vi "ilc.vi"() -> ()   [LabVIEW 2015]
uses:
  Common_RT_ILC/DataTypes/ILCTelemetry.ctl
  Common_RT_ILC/DataTypes/ILCResponses.ctl
  Common_RT_Modbus/DataTypes/ExceptionCodes.ctl
  Common_RT_HPILC/DataTypes/HPResponses.ctl
  Common_RT_HPILC/DataTypes/HPTelemetry.ctl
  Common_RT_HealthAndStatus/RTHealthAndStatus/RTHealthAndStatus.lvclass
  MyHealthAndStatusReadFIFO/MyHealthAndStatusReadFIFO.lvclass
  MyHealthAndStatusWriteFIFO/MyHealthAndStatusWriteFIFO.lvclass
  ModbusFactory/ModbusFactory.lvclass
  SubnetFactory/SubnetFactory.lvclass
  Subnet/DataTypes/SubnetSettings.ctl
  Common_RT_HPILC/DataTypes/HPSettings.ctl
  Common_RT_ILC/DataTypes/ILCSettings.ctl
  Common_RT_Modbus/IModbusFactory/IModbusFactory.lvclass
  ModbusFactory/ModbusFactory.lvclass/ModbusFactory.ctl
  MyHealthAndStatusWriteFIFO/MyHealthAndStatusWriteFIFO.lvclass/MyHealthAndStatusWriteFIFO.ctl
  MyHealthAndStatusReadFIFO/MyHealthAndStatusReadFIFO.lvclass/MyHealthAndStatusReadFIFO.ctl
  Common_RT_HealthAndStatus/RTHealthAndStatus/RTHealthAndStatus.lvclass/RTHealthAndStatus.ctl
  Subnet/Subnet.lvclass/Subnet.ctl
  Common_RT_ILC/ILC/ILC.lvclass/ILC.ctl
  Common_RT_HPILC/HPILC/HPILC.lvclass/HPILC.ctl
  <vilib>/FPGAPlugInAG/cRIO-9038/niLvFpga_Open_cRIO-9038.vi
  <vilib>/rvi/interface/common/dynamic/niFpgaDynamicAddResources.vi
  <vilib>/FPGAPlugInAG/Dynamic/niLvFpga_Abort_Dynamic.vi
  <vilib>/FPGAPlugInAG/Dynamic/niLvFpga_Reset_Dynamic.vi
  <vilib>/FPGAPlugInAG/Dynamic/niLvFpga_Run_Dynamic.vi
  <vilib>/Utility/error.llb/Error Cluster From Error Code.vi
  <vilib>/rvi/errors/niLvFpgaAdjustHostInterfaceError.vi
  <vilib>/FPGAPlugInAG/Dynamic/niLvFpga_Close_Dynamic.vi
  <vilib>/rvi/interface/nirviOpenFPGA/nirviOpenFPGA.xnode
  FPGA Bitfiles/modbus1Port.lvbitx
  FPGA/main.vi
  <vilib>/rvi/interface/nirviMethod/nirviMethod.xnode
  <vilib>/rvi/interface/nirviCloseFPGA/nirviCloseFPGA.xnode
  Common_RT_ILC/RTILC.lvlib
  Common_RT_ILC/ILC/ILC.lvclass
  Common_RT_HPILC/RTHPILC.lvlib
  Common_RT_HPILC/HPILC/HPILC.lvclass
  Common_RT_Modbus/RTModbus.lvlib
  Subnet/Subnet.lvclass
  <vilib>/rvi/errors/niLvFpgaMergeErrorWithErrorCode.vi
  <vilib>/FPGAPlugInAG/Dynamic/niLvFpga_ReadFifo_Dynamic.vi
panel:
  out "Broadcast Counter Error":bool
  out "minMinEncoder":i32
  out "maxMinEncoder":i32
  out "minMaxEncoder":i32
  out "maxMaxEncoder":i32
  out "Exception on Force and Status":bool
  out "minAvgDelta":dbl
  out "maxAvgDelta":dbl
  out "minMaxDelta":i32
  out "maxMaxDelta":i32
  out "minMinDelta":i32
  out "maxMinDelta":i32
  out "MaxDelta":i32(graph)
  out "MinDelta":i32(graph)
  out "AvgDelta":dbl(graph)
  out "avgDelta":dbl
  out "minDelta":i32
  out "maxDelta":i32
  out "minValue":i32
  out "maxValue":i32
  out "Encoder":i32(graph)
  out "Steps":i32
  in  "Stop":bool
  out "HPTelemetry":T1
  out "HPResponses":T2
  in  "Boolean":bool
  out "ILCResponses":T4
  out "ILCTelemetry":T5
  out "Port 1 Status Bits":u64 format="%016b"
  out "error out":errorcluster
  out "Port 1 Frames Received":i64
  out "Port 1 Bytes Received":i64
  out "Port 1 Frames Transmitted":i64
  out "Port 1 Bytes Transmitted":i64
  # "Port 1 = Modbus"
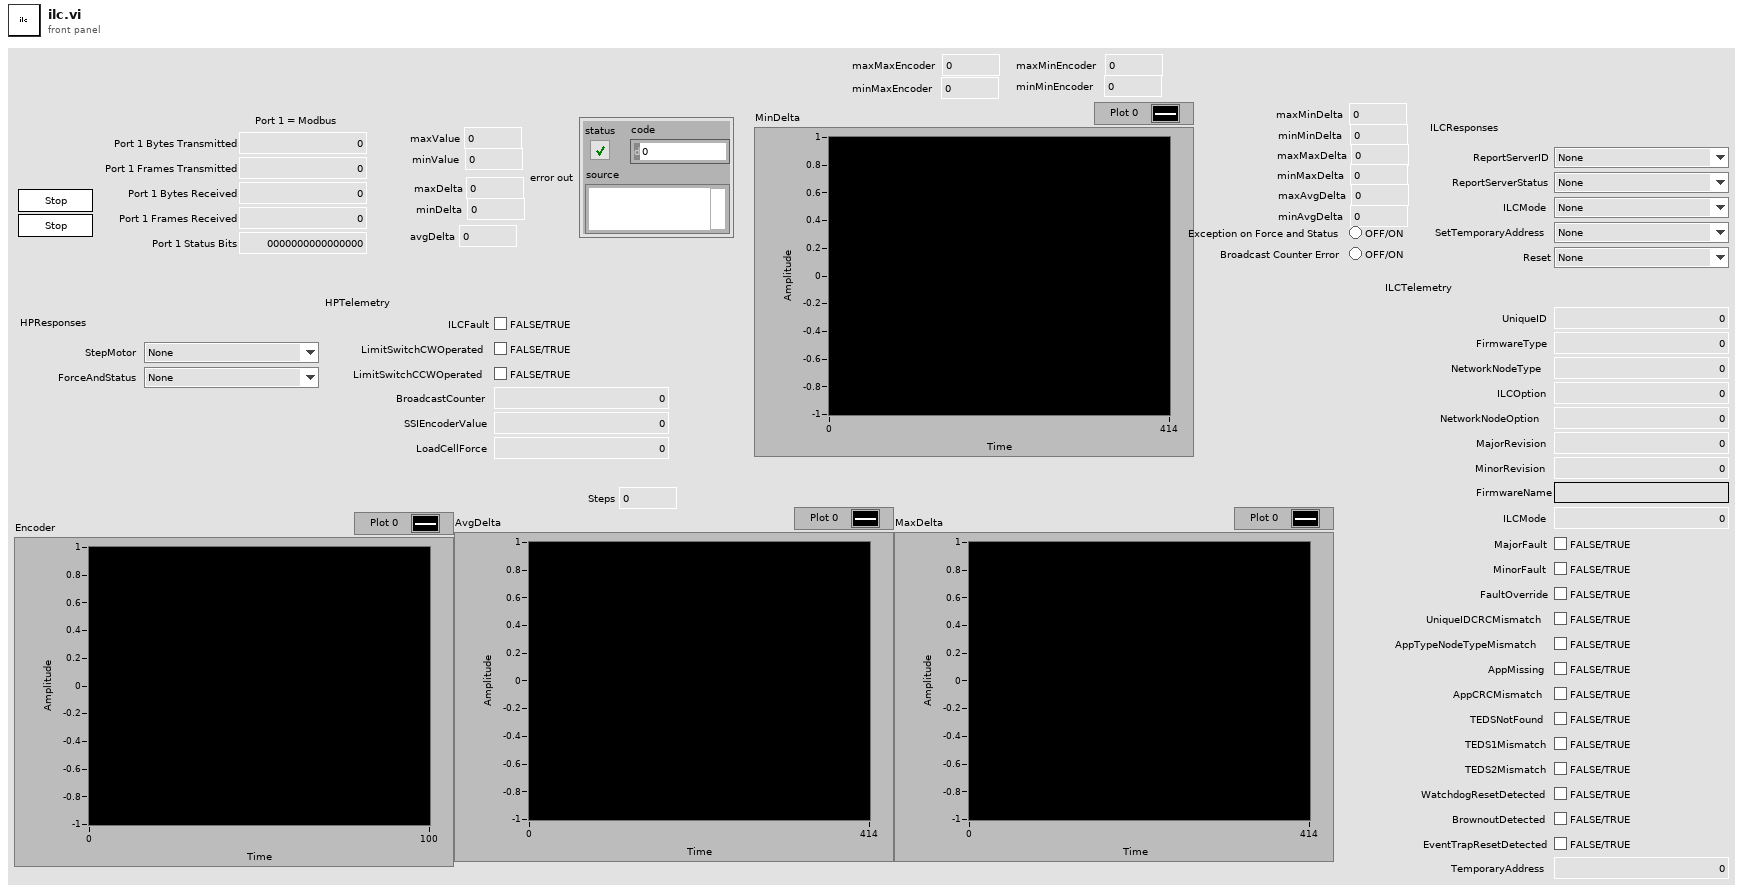
[diagram p1: front panel]
types:
  T1 = typedef "RTHPILC.lvlib/HPTelemetry.ctl" = cluster{"ILCFault":bool, "LimitSwitchCWOperated":bool, "LimitSwitchCCWOperated":bool, "BroadcastCounter":u8, "SSIEncoderValue":i32, "LoadCellForce":sgl}
  T2 = typedef "RTHPILC.lvlib/HPResponses.ctl" = cluster{"StepMotor":T3, "ForceAndStatus":T3}
  T3 = typedef "RTModbus.lvlib/ExceptionCodes.ctl" = enum16{"None", "IllegalFunction", "IllegalDataAddress", "IllegalDataValue", "SlaveDeviceFailure", "Acknowledge", "SlaveDeviceBusy", "NegativeAcknowledge", "MemoryParityError", "GatewayPathUnavailable", "GatewayTargetDeviceFailedToRespond"}
  T4 = typedef "RTILC.lvlib/ILCResponses.ctl" = cluster{"ReportServerID":T3, "ReportServerStatus":T3, "ILCMode":T3, "SetTemporaryAddress":T3, "Reset":T3}
  T5 = typedef "RTILC.lvlib/ILCTelemetry.ctl" = cluster{"UniqueID":u64, "FirmwareType":u8, "NetworkNodeType":u8, "ILCOption":u8, "NetworkNodeOption":u8, "MajorRevision":u8, "MinorRevision":u8, "FirmwareName":string, "ILCMode":u16, "MajorFault":bool, "MinorFault":bool, "FaultOverride":bool, "UniqueIDCRCMismatch":bool, "AppTypeNodeTypeMismatch":bool, "AppMissing":bool, "AppCRCMismatch":bool, "TEDSNotFound":bool, "TEDS1Mismatch":bool, "TEDS2Mismatch":bool, "WatchdogResetDetected":bool, "BrownoutDetected":bool, "EventTrapResetDetected":bool, "TemporaryAddress":u8}
  T6 = typedef "RTHPILC.lvlib/HPSettings.ctl" = cluster{"ILCSettings":T7, "ID":i16, "ReferencePosition":u32}
  T7 = typedef "RTILC.lvlib/ILCSettings.ctl" = cluster{"Subnet":u8, "Address":u8}
  T8 = typedef "SubnetSettings.ctl" = cluster{"HPs":T6[], "ModbusFactory":refnum<class "IModbusFactory.lvclass">, "Port":i32}
  T9 = typedef "SubnetData.ctl" = cluster{"SubnetConstants":T10, "SubnetCommand":T13, "SubnetTelemetry":T14}
  T10 = typedef "SubnetConstants.ctl" = cluster{"Modbus":refnum<class "IModbus.lvclass">, "HPs":refnum<class "HPILC.lvclass">[], "AddressToActuator":T11[]}
  T11 = typedef "ILCIndexData.ctl" = cluster{"ILCTypes":T12, "Index":i32}
  T12 = typedef "ILCTypes.ctl" = enum16{"Undefined", "SAA", "DAA", "HP"}
  T13 = typedef "SubnetCommand.ctl" = cluster{"BroadcastCounter":u8}
  T14 = typedef "SubnetTelemetry.ctl" = cluster{"BytesTransmitted":u32, "FramesTransmitted":u32, "BytesReceived":u32, "FramesReceived":u32, "TxInternalFIFOOverflow":bool, "InvalidInstruction":bool, "WaitForRxFrameTimeout":bool, "StartBitError":bool, "StopBitError":bool, "RxDataFIFOOverflow":bool}
  T15 = typedef "RTHPILC.lvlib/HPData.ctl" = cluster{"HPConstants":T16, "HPCommand":T17, "HPTelemetry":T1, "HPResponses":T2}
  T16 = typedef "RTHPILC.lvlib/HPConstants.ctl" = cluster{"ID":i16, "ReferencePosition":u32}
  T17 = typedef "RTHPILC.lvlib/HPCommand.ctl" = cluster{"Steps":i8}
  T18 = typedef "RTILC.lvlib/ILCData.ctl" = cluster{"Constants":T19, "Command":T20, "Telemetry":T5, "Responses":T4}
  T19 = typedef "RTILC.lvlib/ILCConstants.ctl" = cluster{"Subnet":u8, "Address":u8}
  T20 = typedef "RTILC.lvlib/ILCCommand.ctl" = cluster{"ILCMode":u16, "TemporaryAddress":u8}
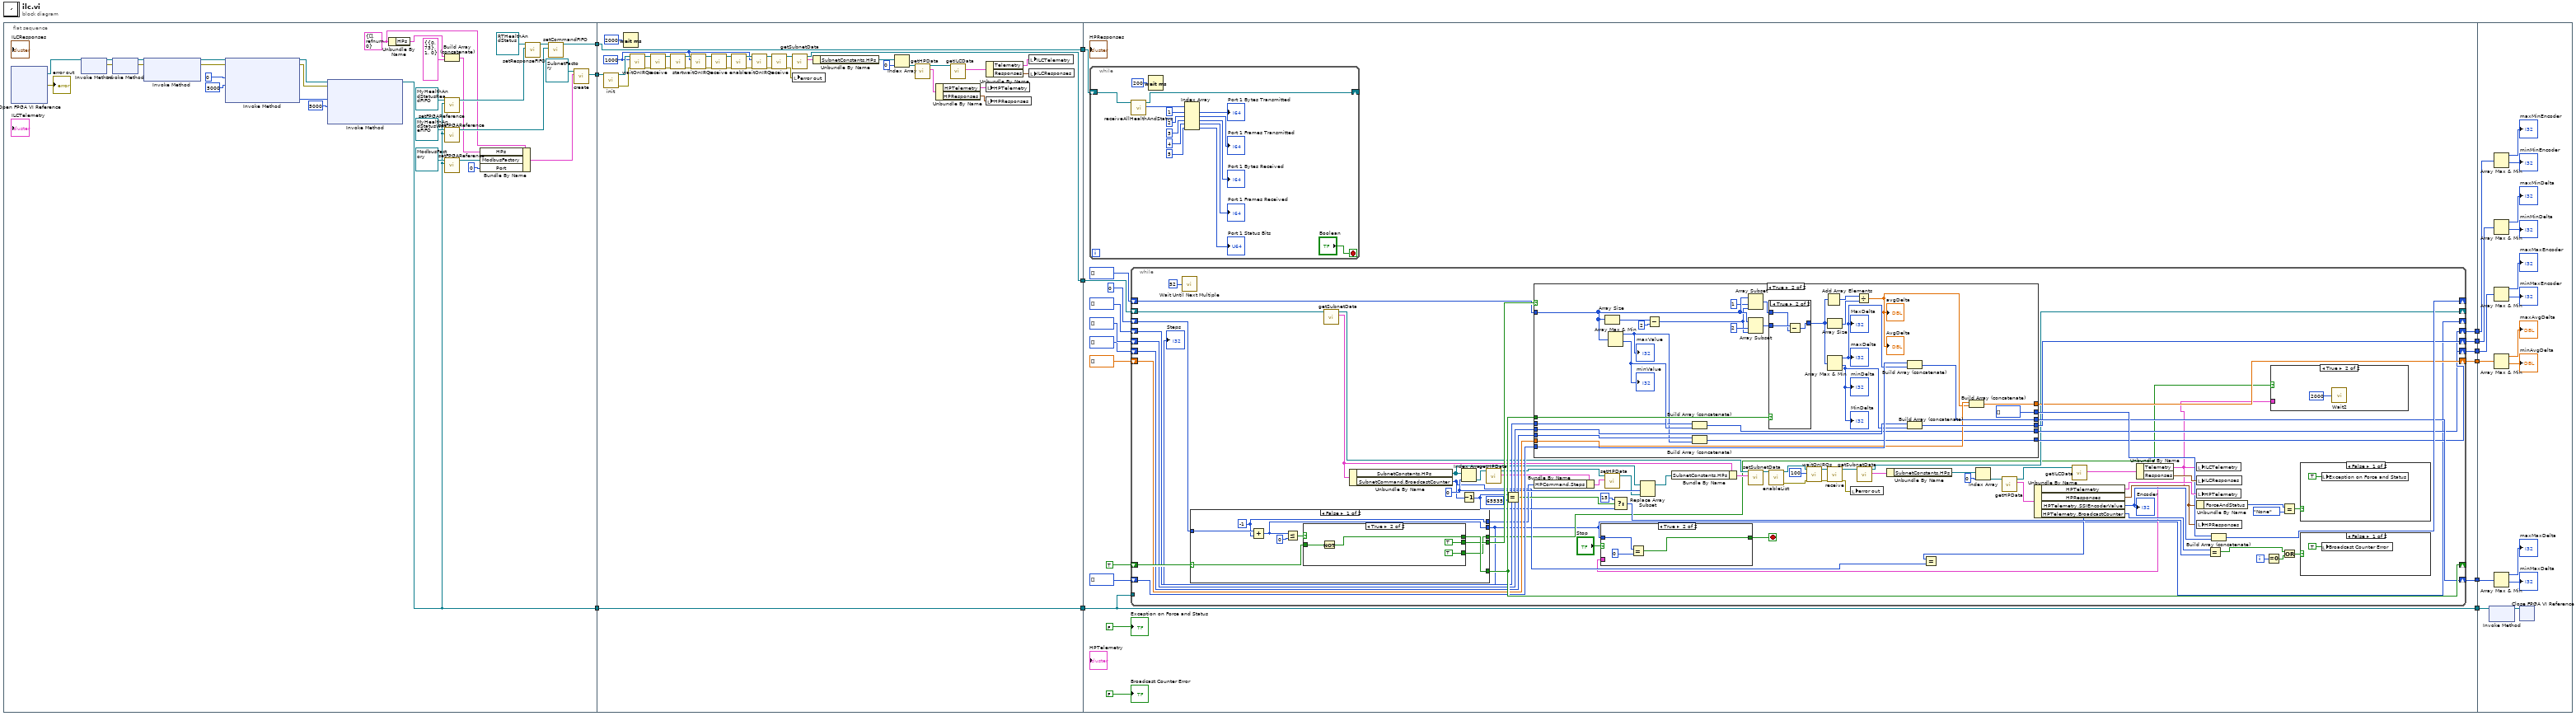
[diagram p0: block diagram]
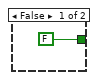
[diagram p5: hidden frame]
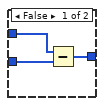
[diagram p7: hidden frame]
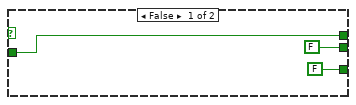
[diagram p8: hidden frame]
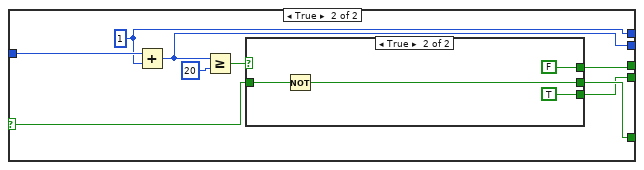
[diagram p9: hidden frame]
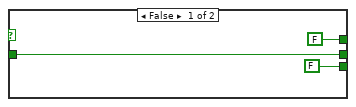
[diagram p10: hidden frame]
diagram:
  n1 = flat-sequence {
    tunnel: [w15] -> w12
    tunnel: [w41] -> w9
    tunnel: [w25] -> w2
    tunnel: w12 -> [w79]
    tunnel: [w79] -> w11
    tunnel: w9 -> [w77]
    tunnel: [w77] -> w8
    tunnel: w2 -> [w76]
    tunnel: [w46] -> w1
    tunnel: w11 -> [w94]
    tunnel: [w94] -> w10
    tunnel: w8 -> [w97]
    tunnel: [w89] -> w7
    tunnel: [w88] -> w6
    tunnel: [w87] -> w5
    tunnel: [w84] -> w4
    tunnel: [w82] -> w3
    tunnel: w1 -> [w81]
    tunnel: w10 -> [w277]
    tunnel: w7 -> [w276]
    tunnel: w6 -> [w273]
    tunnel: w5 -> [w270]
    tunnel: w4 -> [w267]
    tunnel: w3 -> [w264]
    frame #0 {
      w30 = T8 {"HPs"=[], "ModbusFactory"=refnum, "Port"=0} ("SubnetSettings")
      n2 = xnode "Open FPGA VI Reference"() -> ("FPGA VI Reference Out"=w35:refnum<k20>, "error out"=→"error out":errorcluster)  [unwired: 2 in]
      n3 = xnode "Invoke Method"("FPGA VI Reference In"=w35) -> ("FPGA VI Reference Out"=w44:refnum<k20>, "error out"=w36:errorcluster)  [unwired: 1 in]
      n4 = xnode "Invoke Method"("FPGA VI Reference In"=w44, "error in"=w36) -> ("FPGA VI Reference Out"=w17:refnum<k20>, "error out"=w14:errorcluster)
      n5 = xnode "Invoke Method"("FPGA VI Reference In"=w17, "error in"=w14) -> ("FPGA VI Reference Out"=w16:refnum<k20>, "error out"=w13:errorcluster)  [unwired: 1 in]
      n6 = xnode "Invoke Method"("FPGA VI Reference In"=w16, "error in"=w13, "Number of Elements"=u32 0, "Timeout (ms)"=5000) -> ("FPGA VI Reference Out"=w20:refnum<k20>, "error out"=w18:errorcluster, "Elements Remaining"=w21:u32)  [unwired: 1 out]
      n7 = xnode "Invoke Method"("FPGA VI Reference In"=w20, "error in"=w18, "Number of Elements"=w21, "Timeout (ms)"=5000) -> ("FPGA VI Reference Out"=w15:refnum<k20>)  [unwired: 3 out]
      n8 = Unbundle By Name(w30) -> ("HPs"=w32:T6[])
      n9 = Build Array (concatenate)(w32, T6 {"ILCSettings"={"Subnet"=0, "Address"=73}, "ID"=1, "ReferencePosition"=0} ("HPSettings")) -> (w24:T6[])
      n10 = call "setFPGAReference.vi"("FPGAReference"=w15, "MyHealthAndStatusReadFIFO in"=refnum<class "MyHealthAndStatusReadFIFO.lvclass"> refnum ("MyHealthAndStatusReadFIFO.lvclass")) -> ("MyHealthAndStatusReadFIFO out"=w39:refnum<class "MyHealthAndStatusReadFIFO.lvclass">)  [unwired: 9 in]
      n11 = call "setFPGAReference.vi"("FPGAReference"=w15, "MyHealthAndStatusWriteFIFO in"=refnum<class "MyHealthAndStatusWriteFIFO.lvclass"> refnum ("MyHealthAndStatusWriteFIFO.lvclass")) -> ("MyHealthAndStatusWriteFIFO out"=w37:refnum<class "MyHealthAndStatusWriteFIFO.lvclass">)  [unwired: 9 in]
      n12 = call "setFPGAReference.vi"("FPGAReference"=w15, "ModbusFactory in"=refnum<class "ModbusFactory.lvclass"> refnum ("ModbusFactory.lvclass")) -> ("ModbusFactory out"=w28:refnum<class "ModbusFactory.lvclass">)  [unwired: 9 in]
      n13 = Bundle By Name(cluster=w30, "HPs"=w24, "ModbusFactory"=w28, "Port"=0) -> (w27:T8)
      n14 = call "setResponseFIFO.vi"("ReadU32FIFO"=w39, "RTHealthAndStatus in"=refnum<class "RTHealthAndStatus.lvclass"> refnum ("RTHealthAndStatus.lvlib:RTHealthAndStatus.lvclass")) -> ("RTHealthAndStatus out"=w42:refnum<class "RTHealthAndStatus.lvclass">)  [unwired: 9 in]
      n15 = call "setCommandFIFO.vi"("WriteU64FIFO"=w37, "RTHealthAndStatus in"=w42) -> ("RTHealthAndStatus out"=w41:refnum<class "RTHealthAndStatus.lvclass">)  [unwired: 9 in]
      n16 = call "create.vi"("SubnetSettings"=w27, "SubnetFactory in"=refnum<class "SubnetFactory.lvclass"> refnum ("SubnetFactory.lvclass")) -> ("Subnet"=w25:refnum<class "Subnet.lvclass">)  [unwired: 7 in, 2 out]
    }
    frame #1 {
      w59 = 1000 ("Timeout (ms)")
      n17 = call "init.vi"("Subnet in"=w76) -> ("error out"=w72:errorcluster, "Subnet out"=w75:refnum<class "Subnet.lvclass">)  [unwired: 9 in]
      n18 = Wait (ms)(milliseconds to wait=u32 2000) -> ()  [unwired: 1 out]
      n19 = call "waitOnIRQs.vi"("error in (no error)"=w72, "Timeout (ms)"=w59, "Subnet in"=w75) -> ("error out"=w73:errorcluster, "Subnet out"=w74:refnum<class "Subnet.lvclass">)  [unwired: 7 in]
      n20 = call "receive.vi"("error in (no error)"=w73, "Subnet in"=w74) -> ("error out"=w69:errorcluster, "Subnet out"=w71:refnum<class "Subnet.lvclass">)  [unwired: 8 in]
      n21 = call "start.vi"("error in (no error)"=w69, "Subnet in"=w71) -> ("error out"=w68:errorcluster, "Subnet out"=w70:refnum<class "Subnet.lvclass">)  [unwired: 8 in]
      n22 = call "waitOnIRQs.vi"("error in (no error)"=w68, "Timeout (ms)"=w59, "Subnet in"=w70) -> ("error out"=w66:errorcluster, "Subnet out"=w67:refnum<class "Subnet.lvclass">)  [unwired: 7 in]
      n23 = call "receive.vi"("error in (no error)"=w66, "Subnet in"=w67) -> ("error out"=w64:errorcluster, "Subnet out"=w65:refnum<class "Subnet.lvclass">)  [unwired: 8 in]
      n24 = call "enable.vi"("error in (no error)"=w64, "Subnet in"=w65) -> ("error out"=w60:errorcluster, "Subnet out"=w63:refnum<class "Subnet.lvclass">)  [unwired: 8 in]
      n25 = call "waitOnIRQs.vi"("error in (no error)"=w60, "Timeout (ms)"=w59, "Subnet in"=w63) -> ("error out"=w62:errorcluster, "Subnet out"=w61:refnum<class "Subnet.lvclass">)  [unwired: 7 in]
      n26 = call "receive.vi"("error in (no error)"=w62, "Subnet in"=w61) -> ("error out"=w45:errorcluster, "Subnet out"=w58:refnum<class "Subnet.lvclass">)  [unwired: 8 in]
      n27 = call "getSubnetData.vi"("Subnet in"=w58) -> ("SubnetData"=w57:T9, "Subnet out"=w46:refnum<class "Subnet.lvclass">)  [unwired: 9 in]
      n28 = local write "error out"(w45) -> ()
      n29 = Unbundle By Name(w57) -> ("SubnetConstants.HPs"=w56:refnum<class "HPILC.lvclass">[])
      n30 = Index Array(array=w56, index=0) -> (element=w54:refnum<class "HPILC.lvclass">)
      n31 = call "getHPData.vi"("HardPointActuator in"=w54) -> ("HPData"=w50:T15, "HardPointActuator out"=w53:refnum<class "HPILC.lvclass">)  [unwired: 9 in]
      n32 = Unbundle By Name(w50) -> ("HPTelemetry"=w52:T1, "HPResponses"=w51:T2)
      n33 = call "getILCData.vi"("ILC in"=w53) -> ("ILCData"=w47:T18)  [unwired: 9 in, 1 out]
      n34 = Unbundle By Name(w47) -> ("Telemetry"=w49:T5, "Responses"=w48:T4)
      n35 = local write "HPTelemetry"(w52) -> ()
      n36 = local write "HPResponses"(w51) -> ()
      n37 = local write "ILCTelemetry"(w49) -> ()
      n38 = local write "ILCResponses"(w48) -> ()
    }
    frame #2 {
      n39 = while {
        shift-right: [w259] -> _
        shift-left: w97 -> [w260]
        stop <- "Boolean" stop-if-true
        n40 = call "receiveAllHealthAndStatus.vi"("RTHealthAndStatus in"=w260) -> ("Data"=w254:u32[], "RTHealthAndStatus out"=w259:refnum<class "RTHealthAndStatus.lvclass">)  [unwired: 8 in, 1 out]
        n41 = Wait (ms)(milliseconds to wait=u32 200) -> ()  [unwired: 1 out]
        n42 = Index Array(array=w254, index #1=1 ("index"), index #2=2 ("index"), index #3=3 ("index"), index #4=4 ("index"), index #5=5 ("index")) -> (element #1=→"Port 1 Bytes Transmitted":u32, element #2=→"Port 1 Frames Transmitted":u32, element #3=→"Port 1 Bytes Received":u32, element #4=→"Port 1 Frames Received":u32, element #5=→"Port 1 Status Bits":u32)
      }
      n43 = while {
        shift-right: [w98] -> _
        shift-left: 0 -> [w166]
        shift-right: [w152] -> _
        shift-left: TRUE -> [w167]
        tunnel: w94 -> [_]
        shift-right: [w155] -> _
        shift-left: i32[] [] -> [w158]
        shift-right: [w150] -> w88
        shift-left: i32[] [] -> [w151]
        shift-right: [w148] -> w89
        shift-left: i32[] [] -> [w149]
        shift-right: [w146] -> w87
        shift-left: dbl[] [] -> [w147]
        shift-right: [w140] -> w84
        shift-left: i32[] [] -> [w141]
        shift-right: [w138] -> w82
        shift-left: i32[] [] -> [w139]
        shift-right: [w117] -> _
        shift-left: w81 -> [w128]
        i -> [w111]
        stop <- w153 stop-if-true
        w130 = 0 ("index")
        n44 = call "Wait Until Next Multiple"("Count(mSec)"=u32 52) -> ()  [unwired: 1 out]
        n45 = case shown="False" w167 {
          selector: w167 -> [w220 w236]
          tunnel: w166 -> [w222 w239]
          tunnel: [w219 w235] -> w152
          tunnel: [w218 w234] -> w98
          tunnel: [w216 w233] -> w116
          tunnel: [w217 w232] -> w159
          tunnel: [w215 w231] -> w100
          frame False {
            w216 = -1 ("y")
            n46 = Add(x=w222, y=w216) -> (x+y=w218:i32)
            n47 = Less Or Equal?(x=w218, y=0) -> (x <= y?=w221:bool)
            n48 = case shown="True" w221 {
              tunnel: w220 -> [w226 w230]
              tunnel: [w226 w229] -> w219
              tunnel: [FALSE TRUE] -> w217
              tunnel: [FALSE TRUE] -> w215
              frame False {
              }
              frame True {
                n49 = Not(x=w230) -> (.not. x?=w229:bool)
              }
            }
          }
          frame True {
            w233 = 1 ("y")
            n50 = Add(x=w239, y=w233) -> (x+y=w234:i32)
            n51 = Greater Or Equal?(x=w234, y=20) -> (x >= y?=w237:bool)
            n52 = case shown="True" w237 {
              tunnel: w236 -> [w242 w245]
              tunnel: [w242 w246] -> w235
              tunnel: [FALSE TRUE] -> w232
              tunnel: [FALSE FALSE] -> w231
              frame False {
              }
              frame True {
                n53 = Not(x=w245) -> (.not. x?=w246:bool)
              }
            }
          }
        }
        "Steps" <- w98
        n54 = call "getSubnetData.vi"("Subnet in"=w128) -> ("SubnetData"=w127:T9, "Subnet out"=w124:refnum<class "Subnet.lvclass">)  [unwired: 9 in]
        n55 = Unbundle By Name(w127) -> ("SubnetConstants.HPs"=w131:refnum<class "HPILC.lvclass">[], "SubnetCommand.BroadcastCounter"=w103:u8)
        n56 = Index Array(array=w131, index=w130) -> (element=w135:refnum<class "HPILC.lvclass">)
        n57 = Decrement(x=w103) -> (x-1=w106:u8)
        n58 = call "getHPData.vi"("HardPointActuator in"=w135) -> ("HPData"=w134:T15, "HardPointActuator out"=w132:refnum<class "HPILC.lvclass">)  [unwired: 9 in]
        n59 = Equal?(x=w106, y=u16 65535) -> (x = y?=w104:bool)
        n60 = case shown="True" w159 {
          tunnel: w158 -> [w180 w206]
          tunnel: [w180 i32[] []] -> w157
          tunnel: w152 -> [_ w202]
          tunnel: w151 -> [w179 w195]
          tunnel: [w179 w194] -> w150
          tunnel: w149 -> [w178 w193]
          tunnel: [w178 w192] -> w148
          tunnel: w147 -> [w177 w191]
          tunnel: [w177 w190] -> w146
          tunnel: w141 -> [w176 w186]
          tunnel: [w176 w185] -> w140
          tunnel: w139 -> [w175 w183]
          tunnel: [w175 w182] -> w138
          frame False {
          }
          frame True {
            n61 = Array Size(array=w206) -> (size(s)=w201:i32)
            n62 = Array Max & Min(array=w206) -> (max value=w181:i32, min value=w184:i32)  [unwired: 2 out]
            "maxValue" <- w181
            "minValue" <- w184
            n63 = Subtract(x=w201, y=2) -> (x-y=w199:i32)
            n64 = Build Array (concatenate)(w183, w184) -> (w182:i32[])
            n65 = Build Array (concatenate)(w186, w181) -> (w185:i32[])
            n66 = Array Subset(array=w206, index=1, length=w199) -> (w203:i32[])
            n67 = Array Subset(array=w206, index=2, length=w199) -> (w204:i32[])
            n68 = case shown="True" w202 {
              tunnel: w204 -> [w210 w214]
              tunnel: w203 -> [w211 w213]
              tunnel: [w209 w212] -> w198
              frame False {
                n69 = Subtract(x=w211, y=w210) -> (x-y=w209:i32[])
              }
              frame True {
                n70 = Subtract(x=w214, y=w213) -> (x-y=w212:i32[])
              }
            }
            n71 = Add Array Elements(numeric array=w198) -> (sum=w197:i32)
            n72 = Array Size(array=w198) -> (size(s)=w196:i32)
            n73 = Array Max & Min(array=w198) -> (max value=w188:i32, min value=w187:i32)  [unwired: 2 out]
            "maxDelta" <- w188
            "minDelta" <- w187
            "MaxDelta" <- w188
            "MinDelta" <- w187
            n74 = Divide(x=w197, y=w196) -> (x/y=w189:dbl)
            "avgDelta" <- w189
            "AvgDelta" <- w189
            n75 = Build Array (concatenate)(w195, w188) -> (w194:i32[])
            n76 = Build Array (concatenate)(w193, w187) -> (w192:i32[])
            n77 = Build Array (concatenate)(w191, w189) -> (w190:dbl[])
          }
        }
        n78 = Bundle By Name(cluster=w134, "HPCommand.Steps"=w116) -> (w133:T15)
        n79 = call "setHPData.vi"("HPData"=w133, "HardPointActuator in"=w132) -> ("HardPointActuator out"=w129:refnum<class "HPILC.lvclass">)  [unwired: 9 in]
        n80 = Select(t=u16 15, s=w104, f=w106) -> (s? t:f=w107:u16)
        n81 = Replace Array Subset(array=w131, new element=w129, index=w130) -> (w126:refnum<class "HPILC.lvclass">[])
        n82 = Bundle By Name(cluster=w127, "SubnetConstants.HPs"=w126) -> (w125:T9)
        n83 = call "setSubnetData.vi"("SubnetData"=w125, "Subnet in"=w124) -> ("Subnet out"=w123:refnum<class "Subnet.lvclass">)  [unwired: 9 in]
        n84 = call "enableList.vi"("Subnet in"=w123) -> ("error out"=w122:errorcluster, "Subnet out"=w137:refnum<class "Subnet.lvclass">)  [unwired: 9 in]
        n85 = call "waitOnIRQs.vi"("error in (no error)"=w122, "Timeout (ms)"=100, "Subnet in"=w137) -> ("error out"=w112:errorcluster, "Subnet out"=w115:refnum<class "Subnet.lvclass">)  [unwired: 7 in]
        n86 = call "receive.vi"("error in (no error)"=w112, "Subnet in"=w115) -> ("error out"=w113:errorcluster, "Subnet out"=w114:refnum<class "Subnet.lvclass">)  [unwired: 8 in]
        n87 = local write "error out"(w113) -> ()
        n88 = call "getSubnetData.vi"("Subnet in"=w114) -> ("SubnetData"=w121:T9, "Subnet out"=w117:refnum<class "Subnet.lvclass">)  [unwired: 9 in]
        n89 = Unbundle By Name(w121) -> ("SubnetConstants.HPs"=w120:refnum<class "HPILC.lvclass">[])
        n90 = Index Array(array=w120, index=0) -> (element=w118:refnum<class "HPILC.lvclass">)
        n91 = call "getHPData.vi"("HardPointActuator in"=w118) -> ("HPData"=w164:T15, "HardPointActuator out"=w160:refnum<class "HPILC.lvclass">)  [unwired: 9 in]
        n92 = Unbundle By Name(w164) -> ("HPTelemetry"=w163:T1, "HPResponses"=w145:T2, "HPTelemetry.SSIEncoderValue"=w156:i32, "HPTelemetry.BroadcastCounter"=w102:u8)
        "Encoder" <- w156
        n93 = Equal?(x=w102, y=w103) -> ()  [unwired: 1 out]
        n94 = call "getILCData.vi"("ILC in"=w160) -> ("ILCData"=w162:T18)  [unwired: 9 in, 1 out]
        n95 = Unbundle By Name(w162) -> ("Telemetry"=w99:T5, "Responses"=w161:T4)
        n96 = case shown="True" "Stop" {
          tunnel: w98 -> [_ w174]
          tunnel: [FALSE w172] -> w153
          tunnel: w99 -> [_ _]
          frame False {
          }
          frame True {
            n97 = Equal?(x=w174, y=0) -> (x = y?=w172:bool)
          }
        }
        n98 = local write "ILCTelemetry"(w99) -> ()
        n99 = local write "ILCResponses"(w161) -> ()
        n100 = local write "HPTelemetry"(w163) -> ()
        n101 = Unbundle By Name(w145) -> ("ForceAndStatus"=w144:T3)
        n102 = local write "HPResponses"(w145) -> ()
        n103 = Equal?(x=w102, y=w107) -> (x = y?=w101:bool)
        n104 = Build Array (concatenate)(w157, w156) -> (w155:i32[])
        n105 = Equal To 0?(x=w111) -> (x = 0?=w110:bool)
        n106 = case shown="True" w100 {
          tunnel: w99 -> [_ _]
          frame False {
          }
          frame True {
            n107 = call "Wait2"("Count(mSec)"=u32 2000) -> ()  [unwired: 1 out]
          }
        }
        n108 = Equal?(x=w144, y=ExceptionCodes."None") -> (x = y?=w142:bool)
        n109 = Or(x=w101, y=w110) -> (x .or. y?=w109:bool)
        n110 = case shown="False" w142 {
          frame False {
            n111 = local write "Exception on Force and Status"(TRUE ("Boolean 2")) -> ()
          }
          frame True {
          }
        }
        n112 = case shown="False" w109 {
          frame False {
            n113 = local write "Broadcast Counter Error"(TRUE ("Broadcast Counter Error")) -> ()
          }
          frame True {
          }
        }
      }
      "Exception on Force and Status" <- FALSE
      "Broadcast Counter Error" <- FALSE
    }
    frame #3 {
      n114 = xnode "Invoke Method"("FPGA VI Reference In"=w277) -> ("FPGA VI Reference Out"=w278:refnum<k20>)  [unwired: 1 in, 1 out]
      n115 = Array Max & Min(array=w264) -> (max value=→"maxMinEncoder":i32, min value=→"minMinEncoder":i32)  [unwired: 2 out]
      n116 = Array Max & Min(array=w276) -> (max value=→"maxMinDelta":i32, min value=→"minMinDelta":i32)  [unwired: 2 out]
      n117 = Array Max & Min(array=w267) -> (max value=→"maxMaxEncoder":i32, min value=→"minMaxEncoder":i32)  [unwired: 2 out]
      n118 = Array Max & Min(array=w270) -> (max value=→"maxAvgDelta":dbl, min value=→"minAvgDelta":dbl)  [unwired: 2 out]
      n119 = Array Max & Min(array=w273) -> (max value=→"maxMaxDelta":i32, min value=→"minMaxDelta":i32)  [unwired: 2 out]
      n120 = xnode "Close FPGA VI Reference"("FPGA VI Reference In"=w278) -> ()  [unwired: 1 in, 1 out]
    }
  }
